vi "Get Mouse Position.vi"(8 "error in (no error)":errorcluster) -> (0 "error out":errorcluster, 3 "Mouse Position":cluster{"Horizontal":i32, "Vertical":i32})   [LabVIEW 2011]
doc: "This VI will return the <B>Mouse Position</B> relative to the upper left corner of the screen. This VI will get the position regardless of what window has focus.\n\n-------------\nDeveloped by Brian Hoover (hooovahh)"
uses:
  <vilib>/Utility/inputDevices.llb/closeMouse.vi
  <vilib>/Utility/inputDevices.llb/mouseAcquire.vi
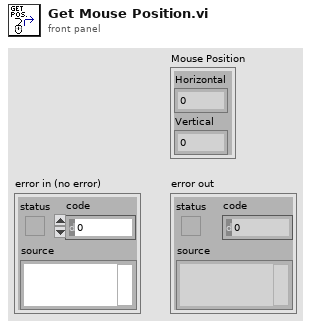
[diagram p1: front panel]
types:
  T1 = cluster{"Horizontal":i32, "Vertical":i32, "Scrolling":i32}
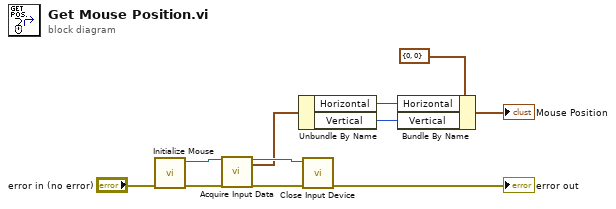
[diagram p0: block diagram]
diagram:
  n1 = call <vilib>:"Initialize Mouse.vi"("error in (no error)"="error in (no error)") -> ("error out"=w8:errorcluster, "device ID"=w11:refnum<k1>)  [unwired: 9 in]
  n2 = call-poly <vilib>:"Acquire Input Data.vi"("device ID"=w11, "error in (no error)"=w8) -> ("device ID"=w10:refnum<k1>, "axis info"=w7:T1, "error out"=w9:errorcluster)  [unwired: 14 in, 1 out]
  n3 = Unbundle By Name(w7) -> ("Horizontal"=w5:i32, "Vertical"=w4:i32)
  n4 = call-poly <vilib>:"Close Input Device.vi"("error in (no error)"=w9, "device ID"=w10) -> ("error out"=→"error out":errorcluster)  [unwired: 8 in]
  n5 = Bundle By Name(cluster=cluster{"Horizontal":i32, "Vertical":i32} {"Horizontal"=0, "Vertical"=0} ("Mouse Position"), "Horizontal"=w5, "Vertical"=w4) -> (→"Mouse Position":cluster{"Horizontal":i32, "Vertical":i32})
